vi "FileDialog.vi"(8 "error in":errorcluster, 10 "default name":string, 11 "start path":path=path "C:/Working copy/tss/HW config/Jung's home.XML") -> (0 "error out":errorcluster, 2 "cancelled":bool=TRUE, 3 "selected path":path)   [LabVIEW 2025, in "Config Tool.lvlib"]
doc: "Opens a Dialog for getting the file Path for the configurationCopyright 2017 National Instruments Corporation\n\nLicensed under the Apache License, Version 2.0 (the \"License\"); you may not use this file except in compliance with the License. You may obtain a copy of the License at http://www.apache.org/licenses/LICENSE-2.0\nUnless required by applicable law or agreed to in writing, software distributed under the License is distributed on an \"AS IS\" BASIS, WITHOUT WARRANTIES OR CONDITIONS OF ANY KIND, either express or implied. See the License for the specific language governing permissions and limitations under the License."
uses:
  Config Tool.lvlib
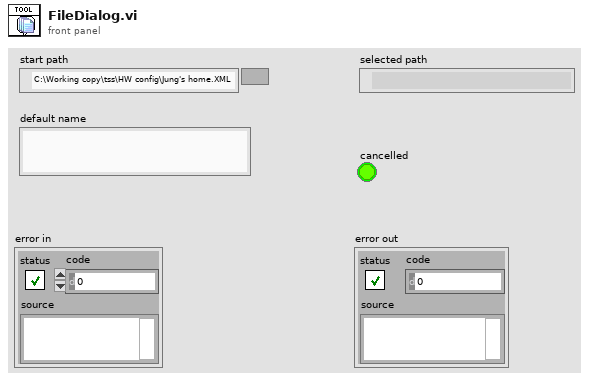
[diagram p1: front panel]
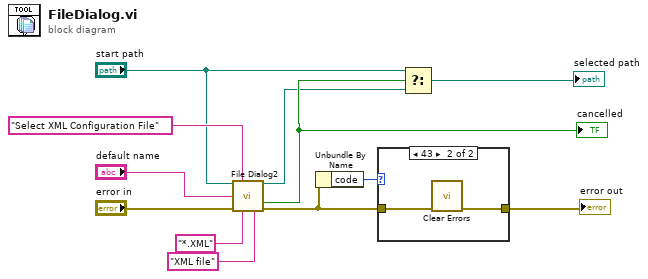
[diagram p0: block diagram]
diagram:
  n1 = call "File Dialog2"("start path"="start path", "prompt"="Select XML Configuration File" ("Prompt"), "default name"="default name", "error in"="error in", "pattern (all files)"="*.XML" ("pattern"), "pattern label"="XML file") -> ("selected path"=w2:path, "cancelled"=w4:bool, "error out"=w6:errorcluster)  [unwired: 6 in, 1 out]
  "cancelled" <- w4
  n2 = Unbundle By Name(w6) -> ("code"=w7:i32)
  n3 = case shown="43" w7 {
    tunnel: w6 -> [w13 w15]
    tunnel: [w13 w14] -> w5
    frame 0, Default {
    }
    frame 43 {
      n4 = call <vilib>:"Clear Errors.vi"("error in (no error)"=w15) -> ("error out"=w14:errorcluster)  [unwired: 5 in, 1 out]
    }
  }
  "error out" <- w5
  n5 = Select(t="start path", s=w4, f=w2) -> (s? t:f=→"selected path":path)
